vi "Parse-2nd-byte.vi"(4 "Error?":bool, 6 "Third Byte Flag":bool=TRUE, 10 "Statustype":string="Polyphonic Key Pressure", 11 "MIDI Parse Data in":T1 {"Current Byte" format="%.0x"; "Running Statusbyte" format="%.0x"; "MIDI-Bytes In" format="%.0x"}) -> (3 "MIDI Parse Data out":T1 {"Current Byte" format="%.0x"; "Running Statusbyte" format="%.0x"; "MIDI-Bytes In" format="%.0x"})   [LabVIEW 2019]
uses:
  Controls/Parser-data.ctl
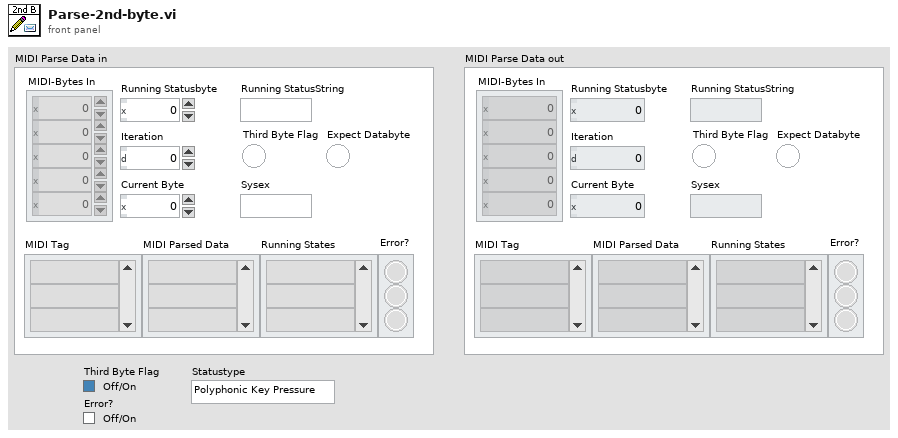
[diagram p1: front panel]
types:
  T1 = typedef "Parser-data.ctl" = cluster{"MIDI-Bytes In":u8[], "MIDI Tag":string[], "MIDI Parsed Data":string[], "Iteration":i32, "Error?":bool[], "Running States":string[], "Running Statusbyte":u8, "Running StatusString":string, "Third Byte Flag":bool, "Current Byte":u8, "Sysex":string, "Expect Databyte":bool}
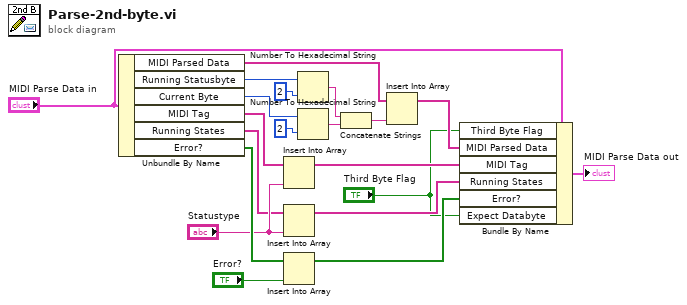
[diagram p0: block diagram]
diagram:
  n1 = Unbundle By Name("MIDI Parse Data in") -> ("MIDI Parsed Data"=w10:string[], "Running Statusbyte"=w4:u8, "Current Byte"=w9:u8, "MIDI Tag"=w13:string[], "Running States"=w15:string[], "Error?"=w18:bool[])
  n2 = Insert Into Array(array=w13, new element="Statustype") -> (w14:string[])  [unwired: 1 in]
  n3 = Insert Into Array(array=w15, new element="Statustype") -> (w17:string[])  [unwired: 1 in]
  n4 = Insert Into Array(array=w18, new element="Error?") -> (w20:bool[])  [unwired: 1 in]
  n5 = Number To Hexadecimal String(1:i16 2 ("width (-)"), 2:w4) -> (0:w6:string)
  n6 = Number To Hexadecimal String(1:i16 2 ("width (-)"), 2:w9) -> (0:w8:string)
  n7 = Concatenate Strings(w6, w8) -> (w11:string)
  n8 = Insert Into Array(array=w10, new element=w11) -> (w12:string[])  [unwired: 1 in]
  n9 = Bundle By Name(cluster="MIDI Parse Data in", "Third Byte Flag"="Third Byte Flag", "MIDI Parsed Data"=w12, "MIDI Tag"=w14, "Running States"=w17, "Error?"=w20, "Expect Databyte"="Third Byte Flag") -> (→"MIDI Parse Data out":T1)
